vi "Mono Filter Wheel.vi"(8 "error in (no error)":errorcluster, 11 "Mono In":refnum<class "Monochromator.lvclass">) -> (0 "error out":errorcluster, 2 "filterWheelPosition":i32)   [LabVIEW 2020, in "Examples.lvlib"]
doc: "This example shows how to get and set the filter wheel position of the mono.\n\nNote: this example will return an error if no internal filter is available."
uses:
  Examples.lvlib
  Classes/Mono/Monochromator.lvclass
panel:
  # "Connector Pane"
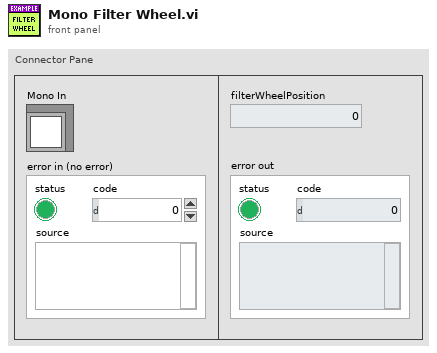
[diagram p1: front panel]
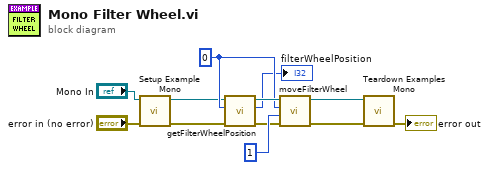
[diagram p0: block diagram]
diagram:
  w8 = 0 ("locationId")
  n1 = call "Setup Example Mono.vi"("error in (no error)"="error in (no error)", "Mono In"="Mono In") -> ("error out"=w3:errorcluster, "Mono Out"=w4:refnum<class "Monochromator.lvclass">)  [unwired: 6 in, 2 out]
  n2 = call "getFilterWheelPosition.vi"("error in (no error)"=w3, "locationId"=w8, "Monochromator in"=w4) -> ("error out"=w5:errorcluster, "position"=→"filterWheelPosition":i32, "Monochromator out"=w9:refnum<class "Monochromator.lvclass">)  [unwired: 6 in]
  n3 = call "moveFilterWheel.vi"("error in (no error)"=w5, "position"=1, "locationId"=w8, "Monochromator in"=w9) -> ("error out"=w1:errorcluster, "Monochromator out"=w2:refnum<class "Monochromator.lvclass">)  [unwired: 4 in, 2 out]
  n4 = call "Teardown Examples Mono.vi"("error in (no error)"=w1, "Monochromator in"=w2) -> ("error out"=→"error out":errorcluster)  [unwired: 9 in]
